vi "DoesScriptContainNull.vi"() -> ()   [LabVIEW 2015]
panel:
  in  "Script Index":i32
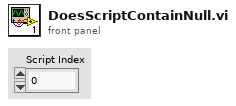
[diagram p1: front panel]
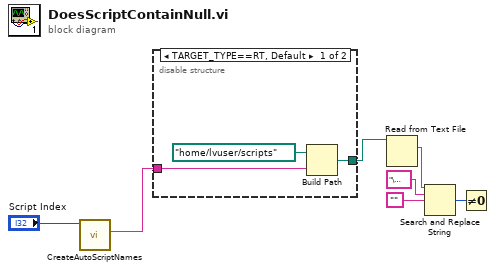
[diagram p0: block diagram]
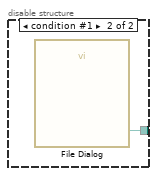
[diagram p2: hidden frame]
diagram:
  n1 = call "CreateAutoScriptNames.vi"("Index"="Script Index") -> ("Concat String"=w1:string)  [unwired: 10 in]
  n2 = disable-structure shown="TARGET_TYPE==RT, Default" {
    disable-tunnel: w1 -> [w10 _]
    disable-tunnel: [w8 w11] -> w4
    frame condition #0 (active) {
      n3 = Build Path(base path=path "/home/lvuser/scripts", name or relative path=w10) -> (appended path=w8:path)
    }
    frame condition #1 {
      n4 = call "File Dialog"() -> ("selected path"=w11:path)  [unwired: 7 in, 8 out]
    }
  }
  n5 = Read from Text File(file (use dialog)=w4) -> (text=w3:string)  [unwired: 1 in, 5 out]
  n6 = Search and Replace String(input string=w3, search string="\u0000" ("regular expression"), replace string="") -> (number of replacements=w5:i32)  [unwired: 5 in, 3 out]
  n7 = Not Equal To 0?(x=w5) -> ()  [unwired: 1 out]
